vi "convert timespec 32 to timespec 64.vi"(11 "timespec 32":cluster{"sec":u32, "nsec":u32}) -> (3 "timespec 64":cluster{"sec":u64, "nsec":u64})   [LabVIEW 2013, in "Linux RT Utilities.lvlib"]
uses:
  Linux RT Utilities.lvlib
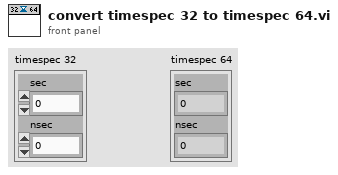
[diagram p1: front panel]
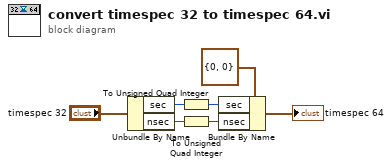
[diagram p0: block diagram]
diagram:
  n1 = Unbundle By Name("timespec 32") -> ("sec"=w5:u32, "nsec"=w4:u32)
  n2 = To Unsigned Quad Integer(1:w5) -> (0:w1:u64)
  n3 = To Unsigned Quad Integer(1:w4) -> (0:w2:u64)
  n4 = Bundle By Name(cluster=cluster{"sec":u64, "nsec":u64} {"sec"=0, "nsec"=0} ("timespec"), "sec"=w1, "nsec"=w2) -> (→"timespec 64":cluster{"sec":u64, "nsec":u64})
